vi "Read Array Delim.vi"(8 "error in (no error)":errorcluster, 11 "Config Data in":refnum<class "Config Data.lvclass">) -> (0 "error out":errorcluster, 2 "Array Delim":string=",", 3 "Config Data out":refnum<class "Config Data.lvclass">)   [LabVIEW 2016, in "Config Data.lvclass"]
uses:
  Config Data.lvclass
  Config Data.lvclass/Config Data.ctl
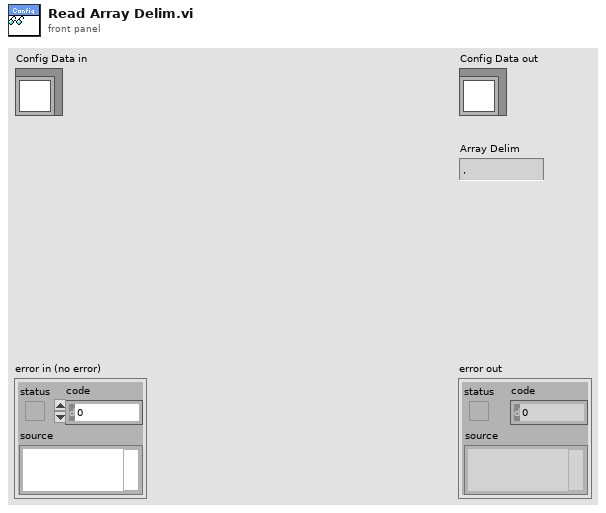
[diagram p1: front panel]
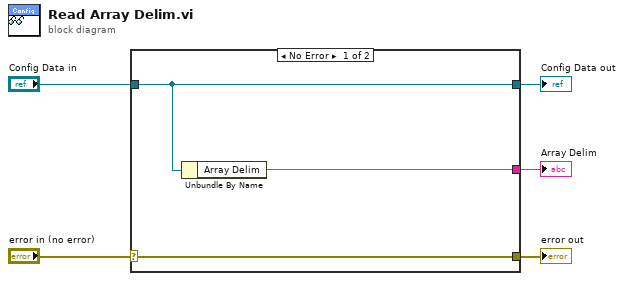
[diagram p0: block diagram]
diagram:
  n1 = case shown="No Error" "error in (no error)" {
    selector: "error in (no error)" -> [w8 w9]
    tunnel: [w8 w9] -> w4
    tunnel: [w7 w10] -> w2
    tunnel: "Config Data in" -> [w7 w10]
    tunnel: [w6 _] -> w1
    frame No Error {
      n2 = Unbundle By Name(w7) -> ("Array Delim"=w6:string)
    }
    frame Error {
    }
  }
  "error out" <- w4
  "Config Data out" <- w2
  "Array Delim" <- w1
